vi "Cam_info.vi"() -> (2 "All Cameras":string[](array[string]), 3 "Array 2":string[](array[string]))   [LabVIEW 2022 SP3]
uses:
  <vilib>/vision/driver/IMAQdx.llb/IMAQdx Attribute Type.ctl
  <vilib>/userdefined/High Color/IMAQdx.ctl
  <vilib>/vision/driver/IMAQdx.llb/IMAQdx Attribute Visibility.ctl
  <vilib>/vision/driver/IMAQdx.llb/IMAQdx Camera Control Mode.ctl
  <vilib>/vision/driver/NI_Vision_Acquisition_Software.lvlib
  <resource>/objmgr/imaqdx.rc
panel:
  out "Array 3":T1(array[cluster])
  out "InterfaceName":string="Camera1"
  out "output cluster":T2
  out "DeviceID":string
  out "DisplayName":string
  out "error out":errorcluster
  out "IMAQdx Session":T3
  in  "error in (no error)":errorcluster
  out "Attribute Information Array":T5(array[cluster])
  out "Array":cluster{"InterfaceName":string, i32}[](array[cluster])
  out "Camera Information Array":T6(array[cluster]) {"BusType" format="%x"; "SerialNumberLow" format="%.0x"; "SerialNumberHigh" format="%.0x"}
  in  "Connected Only? (Yes)":bool=TRUE
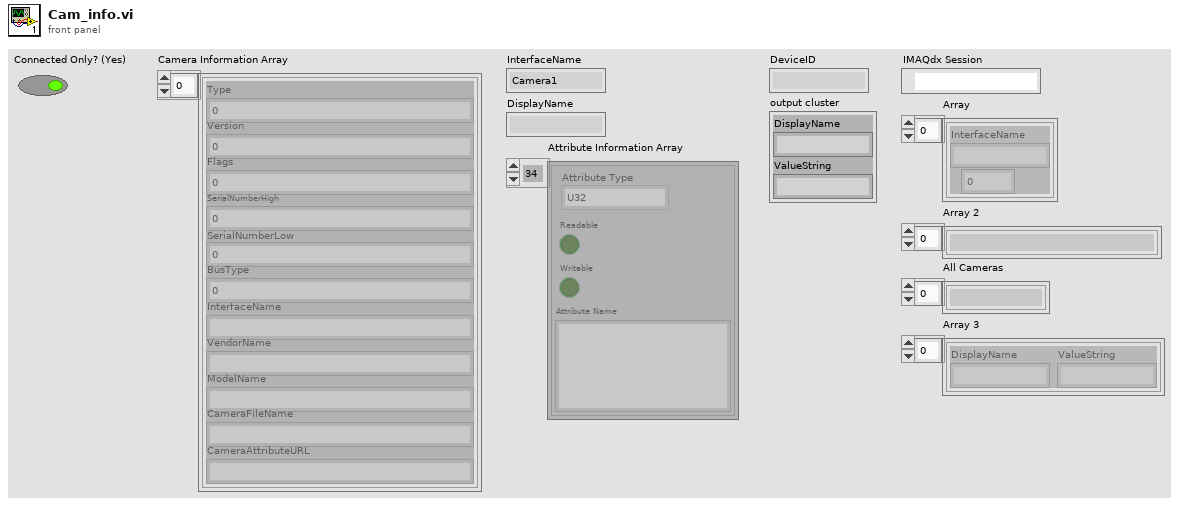
[diagram p1: front panel]
types:
  T1 = cluster{"DisplayName":string, "ValueString":string}[]
  T2 = cluster{"DisplayName":string, "ValueString":string}
  T3 = typedef "IMAQdx.ctl" = refnum<k21>
  T4 = typedef "NI_Vision_Acquisition_Software.lvlib/IMAQdx Attribute Type.ctl" = enum32{"U32", "I64", "DBL", "String", "Enum", "Bool", "Command"}
  T5 = cluster{"Attribute Type":T4, "Readable":bool, "Writable":bool, "Attribute Name":string}[]
  T6 = cluster{"Type":u32, "Version":u32, "Flags":u32, "SerialNumberHigh":u32, "SerialNumberLow":u32, "BusType":u32, "InterfaceName":string, "VendorName":string, "ModelName":string, "CameraFileName":string, "CameraAttributeURL":string}[]
  T7 = typedef "NI_Vision_Acquisition_Software.lvlib/IMAQdx Camera Control Mode.ctl" = enum32{"Controller", "Listener"}
  T8 = typedef "NI_Vision_Acquisition_Software.lvlib/IMAQdx Attribute Visibility.ctl" = enum32{"Simple", "Intermediate", "Advanced"}
  T9 = cluster{"Attribute Type":T4, "Readable":bool, "Writable":bool, "Attribute Name":string}
  T10 = cluster{"InterfaceName":string, "ValueString":string}
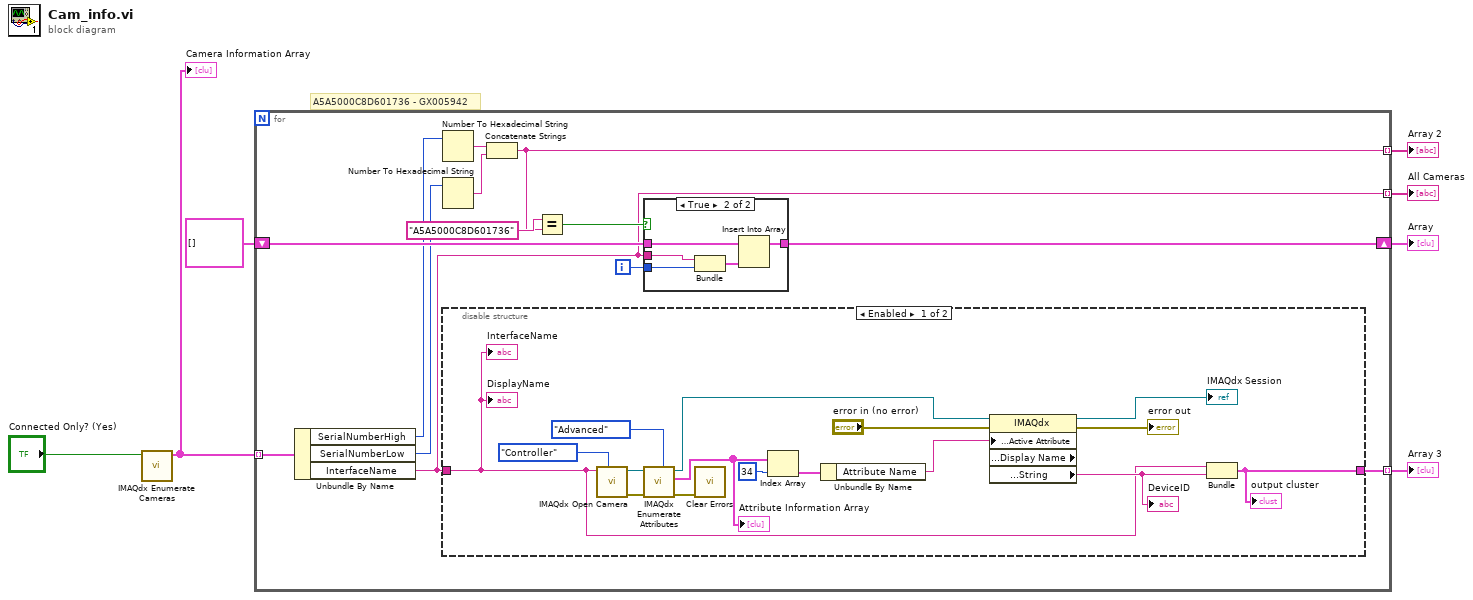
[diagram p0: block diagram]
diagram:
  # "A5A5000C8D601736 - GX005942"
  n1 = call <vilib>:"IMAQdx Enumerate Cameras.vi"("Connected Only? (Yes)"="Connected Only? (Yes)") -> ("Camera Information Array"=w6:T6)  [unwired: 9 in, 1 out]
  "Camera Information Array" <- w6
  n2 = for {
    tunnel: w6 -> [w20] mode=indexing
    shift-right: [w17] -> w3
    shift-left: cluster{"InterfaceName":string, i32}[] [] -> [w16]
    tunnel: [w8] -> w4 mode=indexing
    tunnel: [w10] -> w2 mode=indexing
    tunnel: [w11] -> w1 mode=indexing
    i -> [w18]
    n3 = Unbundle By Name(w20) -> ("SerialNumberHigh"=w13:u32, "SerialNumberLow"=w12:u32, "InterfaceName"=w10:string)
    n4 = Number To Hexadecimal String(2:w13) -> (0:w15:string)  [unwired: 1 in]
    n5 = Number To Hexadecimal String(2:w12) -> (0:w14:string)  [unwired: 1 in]
    n6 = disable-structure shown="Enabled" {
      disable-tunnel: w10 -> [w21 _]
      disable-tunnel: [w23 _] -> w11
      frame Enabled {
        n7 = call <vilib>:"IMAQdx Open Camera.vi"("Camera Control Mode"=IMAQdx_Camera_Control_Mode."Controller", "Session In"=w21) -> ("error out"=w25:errorcluster, "Session Out"=w32:T3)  [unwired: 8 in]
        n8 = call <vilib>:"IMAQdx Enumerate Attributes.vi"("Visibility"=IMAQdx_Attribute_Visibility."Advanced", "error in"=w25, "Session In"=w32) -> ("error out"=w24:errorcluster, "Attribute Information Array"=w36:T5, "Session Out"=w27:T3)  [unwired: 6 in]
        "Attribute Information Array" <- w36
        n9 = call <vilib>:"Clear Errors.vi"("error in (no error)"=w24) -> ()  [unwired: 5 in, 2 out]
        n10 = Index Array(array=w36, index=34) -> (element=w34:T9)
        n11 = Unbundle By Name(w34) -> ("Attribute Name"=w31:string)
        n12 = property class="IMAQdx" props=["Camera Attributes:Active Attribute", "Camera Attributes:Display Name", "Camera Attributes:Value:String"](reference=w27, error in="error in (no error)", "Camera Attributes:Active Attribute"=w31) -> (reference out=→"IMAQdx Session":T3, error out=→"error out":errorcluster, "Camera Attributes:Value:String"=w28:string)  [unwired: 1 out]
        "DeviceID" <- w28
        n13 = Bundle("InterfaceName"=w21, "ValueString"=w28) -> (w23:T10)  [unwired: 1 in]
        "output cluster" <- w23
        "DisplayName" <- w21
        "InterfaceName" <- w21
      }
      frame Disabled {
      }
    }
    n14 = Concatenate Strings(w15, w14) -> (w8:string)
    n15 = Equal?(x="A5A5000C8D601736" ("decimal integer string"), y=w8) -> (x = y?=w19:bool)
    n16 = case shown="True" w19 {
      tunnel: w10 -> [_ w42]
      tunnel: w18 -> [_ w41]
      tunnel: [w37 w40] -> w17
      tunnel: w16 -> [w37 w39]
      frame False {
      }
      frame True {
        n17 = Bundle("InterfaceName"=w42, w41) -> (w38:cluster{"InterfaceName":string, i32})  [unwired: 1 in]
        n18 = Insert Into Array(array=w39, new element=w38) -> (w40:cluster{"InterfaceName":string, i32}[])  [unwired: 1 in]
      }
    }
  }
  "Array" <- w3
  "All Cameras" <- w2
  "Array 2" <- w4
  "Array 3" <- w1
